vi "Tosca-Set Grating Property.vi"(0 "Grating in":T1, 5 "value":dbl, 7 "property":string) -> (4 "Grating out":T1)   [LabVIEW 2020]
uses:
  Tosca-Grating.ctl
  Tosca-Grating Type.ctl
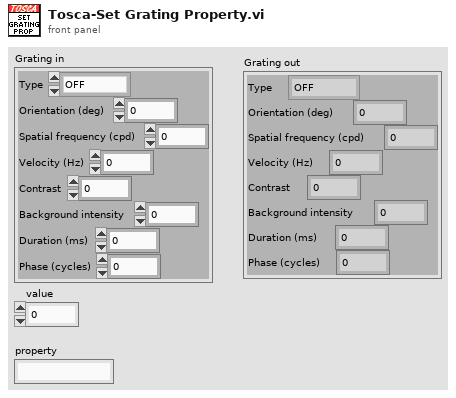
[diagram p1: front panel]
types:
  T1 = typedef "Tosca-Grating.ctl" = cluster{"Type":T2, "Orientation (deg)":dbl, "Spatial frequency (cpd)":dbl, "Velocity (Hz)":dbl, "Contrast":dbl, "Background intensity":dbl, "Duration (ms)":dbl, "Phase (cycles)":dbl}
  T2 = typedef "Tosca-Grating Type.ctl" = enum16{"OFF", "Square", "Sine"}
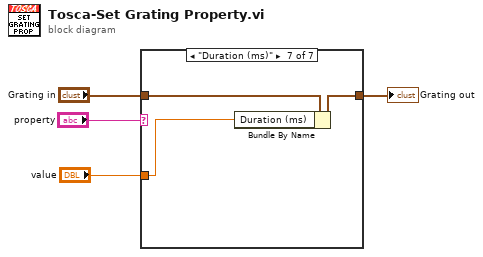
[diagram p0: block diagram]
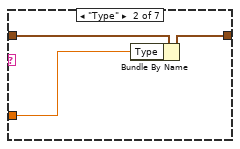
[diagram p3: hidden frame]
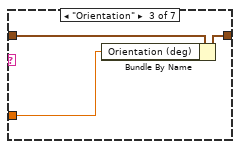
[diagram p4: hidden frame]
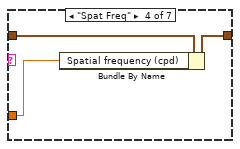
[diagram p5: hidden frame]
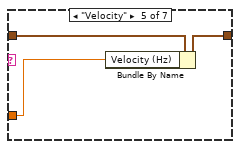
[diagram p6: hidden frame]
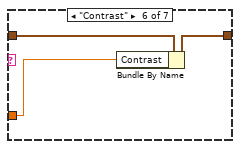
[diagram p7: hidden frame]
diagram:
  n1 = case shown="\"Duration (ms)\"" "property" {
    tunnel: "Grating in" -> [w5 w8 w11 w14 w17 w20 w23]
    tunnel: [w5 w7 w10 w13 w16 w19 w22] -> w2
    tunnel: "value" -> [_ w6 w9 w12 w15 w18 w21]
    frame "", Default {
    }
    frame "Type" {
      n2 = Bundle By Name(cluster=w8, "Type"=w6) -> (w7:T1)
    }
    frame "Orientation" {
      n3 = Bundle By Name(cluster=w11, "Orientation (deg)"=w9) -> (w10:T1)
    }
    frame "Spat Freq" {
      n4 = Bundle By Name(cluster=w14, "Spatial frequency (cpd)"=w12) -> (w13:T1)
    }
    frame "Velocity" {
      n5 = Bundle By Name(cluster=w17, "Velocity (Hz)"=w15) -> (w16:T1)
    }
    frame "Contrast" {
      n6 = Bundle By Name(cluster=w20, "Contrast"=w18) -> (w19:T1)
    }
    frame "Duration (ms)" {
      n7 = Bundle By Name(cluster=w23, "Duration (ms)"=w21) -> (w22:T1)
    }
  }
  "Grating out" <- w2
